vi "DAQ testing.vi"() -> ()   [LabVIEW 2014]
uses:
  <vilib>/DAQmx/read.llb/DAQmx Read (Analog 2D DBL NChan NSamp).vi
  <vilib>/DAQmx/create/channels.llb/DAQmx Create Channel (AI-Voltage-Basic).vi
  <vilib>/DAQmx/configure/timing.llb/DAQmx Timing (Sample Clock).vi
  <vilib>/DAQmx/miscellaneous.llb/DAQmx Fill In Error Info.vi
  <resource>/objmgr/daqmx.rc
panel:
  in  "milliseconds to wait":u32=100
  out "data 2":dbl[][](array[numeric]) format="%0.2f"
  out "x-y":dbl
  out "data":dbl[](array[numeric]) format="%0.2f"
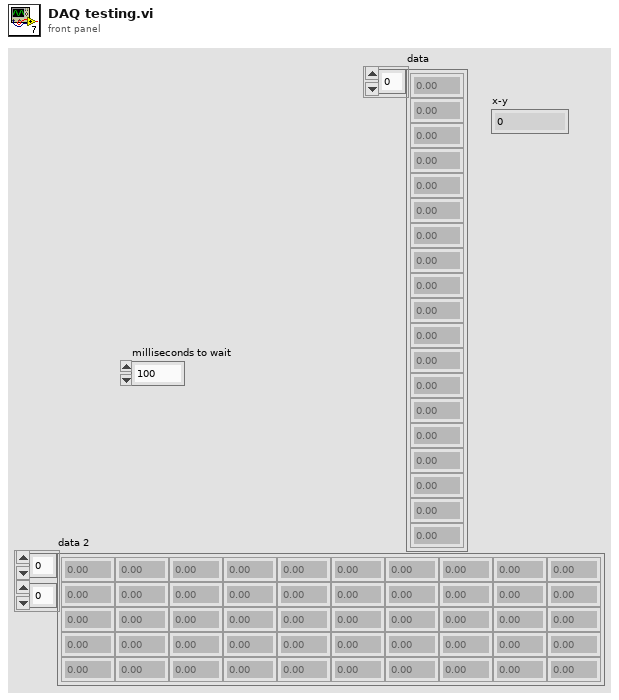
[diagram p1: front panel]
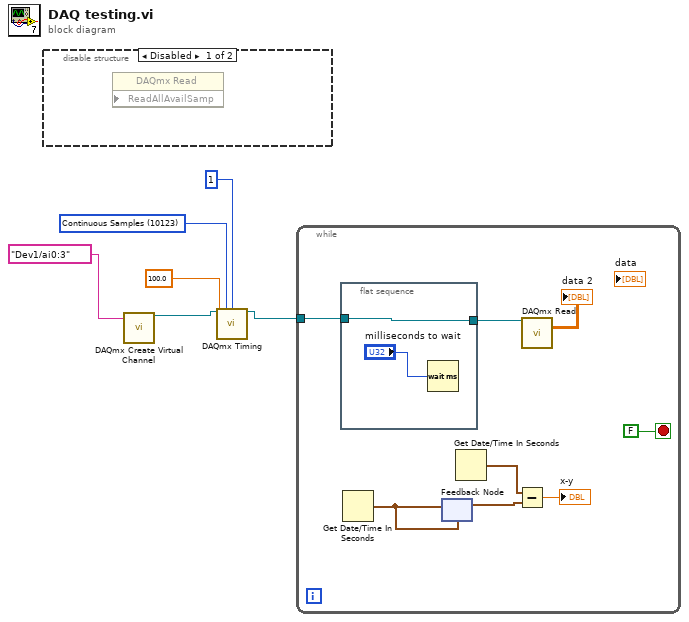
[diagram p0: block diagram]
diagram:
  w3 = 10123 items=["Finite Samples"=10178, "Continuous Samples"=10123, "Hardware Timed Single Point"=12522] ("sample mode")
  n1 = disable-structure shown="Disabled" {
    frame Disabled {
      n2 = property class="DAQmx Read" props=["ReadAllAvailSamp"]() -> ()  [unwired: 3 in, 2 out]
    }
    frame Enabled {
    }
  }
  n3 = call-poly <vilib>:"DAQmx Create Virtual Channel.vi"("physical channels"=tag "Dev1/ai0:3") -> ("task out"=w5:refnum<k21>)  [unwired: 13 in, 1 out]
  n4 = call-poly <vilib>:"DAQmx Timing.vi"("task/channels in"=w5, "sample mode"=w3, "samples per channel"=1, "rate"=100.0) -> ("task out"=w4:refnum<k21>)  [unwired: 10 in, 1 out]
  n5 = while {
    tunnel: w4 -> [w12]
    stop <- FALSE stop-if-true
    n6 = flat-sequence {
      tunnel: [w15] -> w13
      tunnel: w12 -> [w15]
      frame #0 {
        n7 = Wait (ms)(milliseconds to wait="milliseconds to wait") -> ()  [unwired: 1 out]
      }
    }
    n8 = Get Date/Time In Seconds() -> (seconds since 1Jan1904=w11:timestamp)
    n9 = feedback-in #1(w11) -> ()
    n10 = feedback #1(w11) -> (w10:timestamp)
    n11 = Get Date/Time In Seconds() -> (seconds since 1Jan1904=w9:timestamp)
    n12 = Subtract(x=w9, y=w10) -> (x-y=→"x-y":dbl)
    n13 = call-poly <vilib>:"DAQmx Read.vi"("task/channels in"=w13) -> ("data"=→"data 2":dbl[][])  [unwired: 12 in, 2 out]
  }
